vi "log message.vi"(8 "error in (no error)":errorcluster, 9 "message type":string(combo)="[INFO]", 10 "Message to log":string, 11 "Error log in":refnum<class "Error log.lvclass">) -> (0 "error out":errorcluster, 3 "Error log out":refnum<class "Error log.lvclass">)   [LabVIEW 2018, in "Error log.lvclass"]
uses:
  Error log.lvclass
  C:/Users/Denis/Desktop/S4CCS/S4CCS/Log File/CCS_Log File.lvclass
  <vilib>/Utility/error.llb/DialogType.ctl
  Log File/CCS_Log File.lvclass/CCS_Log File.ctl
  Log File/CCS_Log File.lvclass
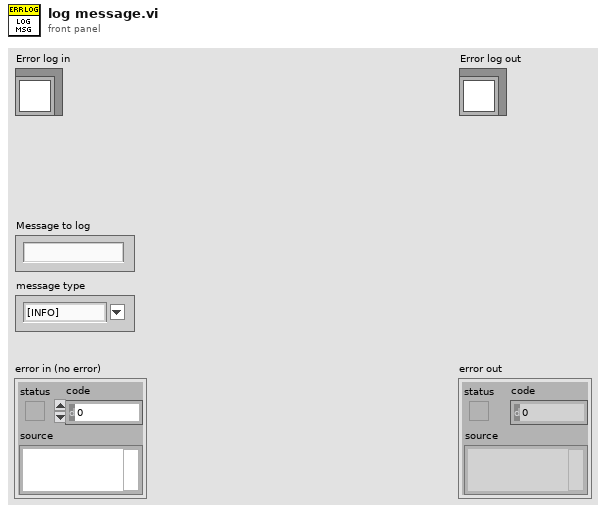
[diagram p1: front panel]
types:
  T1 = typedef "DialogType.ctl" = u16
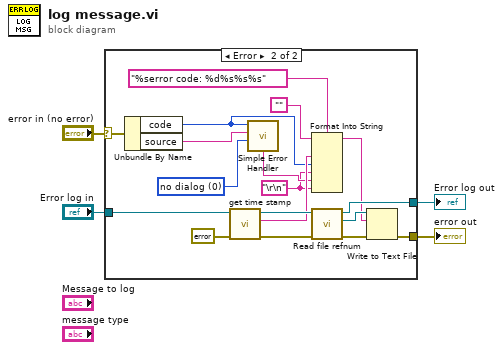
[diagram p0: block diagram]
diagram:
  n1 = case shown="Error" "error in (no error)" {
    selector: "error in (no error)" -> [w6 w15]
    tunnel: [w6 w24] -> w2
    tunnel: "Error log in" -> [w5 w23]
    tunnel: [w5 w18] -> w1
    frame No Error {
    }
    frame Error {
      w7 = "\r\n"
      w16 = T1 0 items=["no dialog", "OK message", "continue or stop message", "OK message + warnings", "continue/stop + warnings"] ("type of dialog (OK msg:1)")
      n2 = Unbundle By Name(w15) -> ("code"=w8:i32, "source"=w14:string)
      n3 = call "get time stamp.vi"("error in (no error)"=errorcluster {"status"=FALSE, "code"=0, "source"=""}, "Log File in"=w23) -> ("error out"=w22:errorcluster, "time stamp"=w12:string, "Log File out"=w19:refnum<class "Error log.lvclass">)  [unwired: 7 in]
      n4 = call <vilib>:"Simple Error Handler.vi"("error code (no error:0)"=w8, "error source (\" \")"=w14, "type of dialog (OK msg:1)"=w16) -> ("message"=w11:string)  [unwired: 2 in, 4 out]
      n5 = Format Into String(format string="%serror code: %d%s%s%s", initial string="", w12, w8, w7, w11, w7) -> (resulting string=w9:string)  [unwired: 1 in, 1 out]
      n6 = call "Read file refnum.vi"("error in (no error)"=w22, "Log File in"=w19) -> ("error out"=w21:errorcluster, "file refnum"=w20:refnum<file>, "Log File out"=w18:refnum<class "Error log.lvclass">)  [unwired: 7 in]
      n7 = Write to Text File(file (use dialog)=w20, text=w9, error in=w21) -> (error out=w24:errorcluster)  [unwired: 1 in, 2 out]
    }
  }
  "error out" <- w2
  "Error log out" <- w1
